vi "Factory.vi"(4 "Use LCD?":bool, 5 "Recycle?":bool, 6 "Reader":T2, 7 "Scan Setup Mode":T1, 8 "error in":errorcluster, 9 "Scanner":T3, 10 "Path":path, 11 "Recycle old Scan Driver in":refnum<class "Scan Driver.lvclass">) -> (0 "error out":errorcluster, 3 "Scan Driver out":refnum<class "Scan Driver.lvclass">)   [LabVIEW 2009, in "Scan Driver.lvclass"]
doc: "Construct a new Scan Driver instance using the given parameters, load one from a file, or recycle an old one."
uses:
  Scan Driver.lvclass
  Scanner List.ctl
  Reader List.ctl
  Scan Setup Mode.ctl
  Scan Driver.lvclass/Scan Driver.ctl
  Scanners/Scanner/Scanner.lvclass
  Instruments/Spectrometer/Spectrometer Triax 550.lvclass
  Instruments/Magnet/Power Supply/Power Supply.lvclass
  Instruments/Pulse Gen/Pulse Generator.lvclass
  Instruments/Function Generator/Function Generator.lvclass
  Instruments/Microwave/Microwave.lvclass
  Instruments/Translation Stages/Translation Stages.lvclass
  Instruments/Spectrometer Digikröm/Spectrometer Digikröm.lvclass
  Instruments/Spectrometer iHR320/Spectrometer iHR320.lvclass
  Instruments/Varian Magnet/Varian Magnet.lvclass
  Instruments/Analog Output/Analog Output.lvclass
  Instruments/Photon Counter/Photon Counter SR400.lvclass
  Instruments/Lockin/Lockin SR830.lvclass
  Instruments/Utility Classes/Dummy/Dummy.lvclass
  Instruments/DAQ/DAQmx Analog.lvclass
  Readers/Reader/Reader.lvclass
  Readers/PC Reader/PC Reader.lvclass
  File IO/File IO.lvclass
  Instruments/LCD/LCD Retarder.lvclass
  Readers/LCD Reader/LCD Reader.lvclass
  Scanners/Dummy Scan/Dummy Scan.lvclass
  Instruments/Magnet/Temperature Controller/Temperature Controller.lvclass
  Instruments/Fluke Multimeter/Fluke Multimeter.lvclass
  Instruments/Power Meter/Power Meter.lvclass
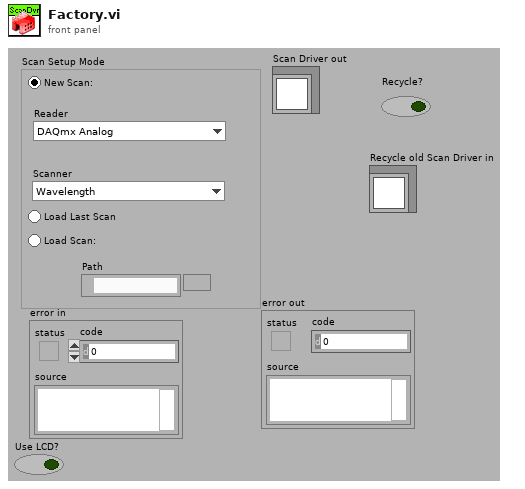
[diagram p1: front panel]
types:
  T1 = typedef "Scan Driver.lvclass/Scan Setup Mode.ctl" = enum32{"New Scan", "Load Last Scan", "Load Scan:"}
  T2 = typedef "Scan Driver.lvclass/Reader List.ctl" = enum16{"DAQmx Analog", "Dummy", "Lockin SR830", "Photon Counter", "Multimeter", "Power Meter", "Temperature Control"}
  T3 = typedef "Scan Driver.lvclass/Scanner List.ctl" = enum16{"Wavelength", "Wavelength Digikröm", "Wavelength iHR320", "Magnetic Field", "Continuous", "Pulse Gen Scan", "Pulse Gen Basic Scan", "Function Gen Scan", "Microwave Freq Scan", "Translation Stage Scan", "Dummy Scan", "Varian Magnet Scan", "Varian Continuous Scan", "Analog Output Scan"}
  T4 = typedef "Scanner.lvclass/Range.ctl" = cluster{"xi":dbl, "xf":dbl, "dx":dbl, "Return to...?":bool, "Return to":dbl}
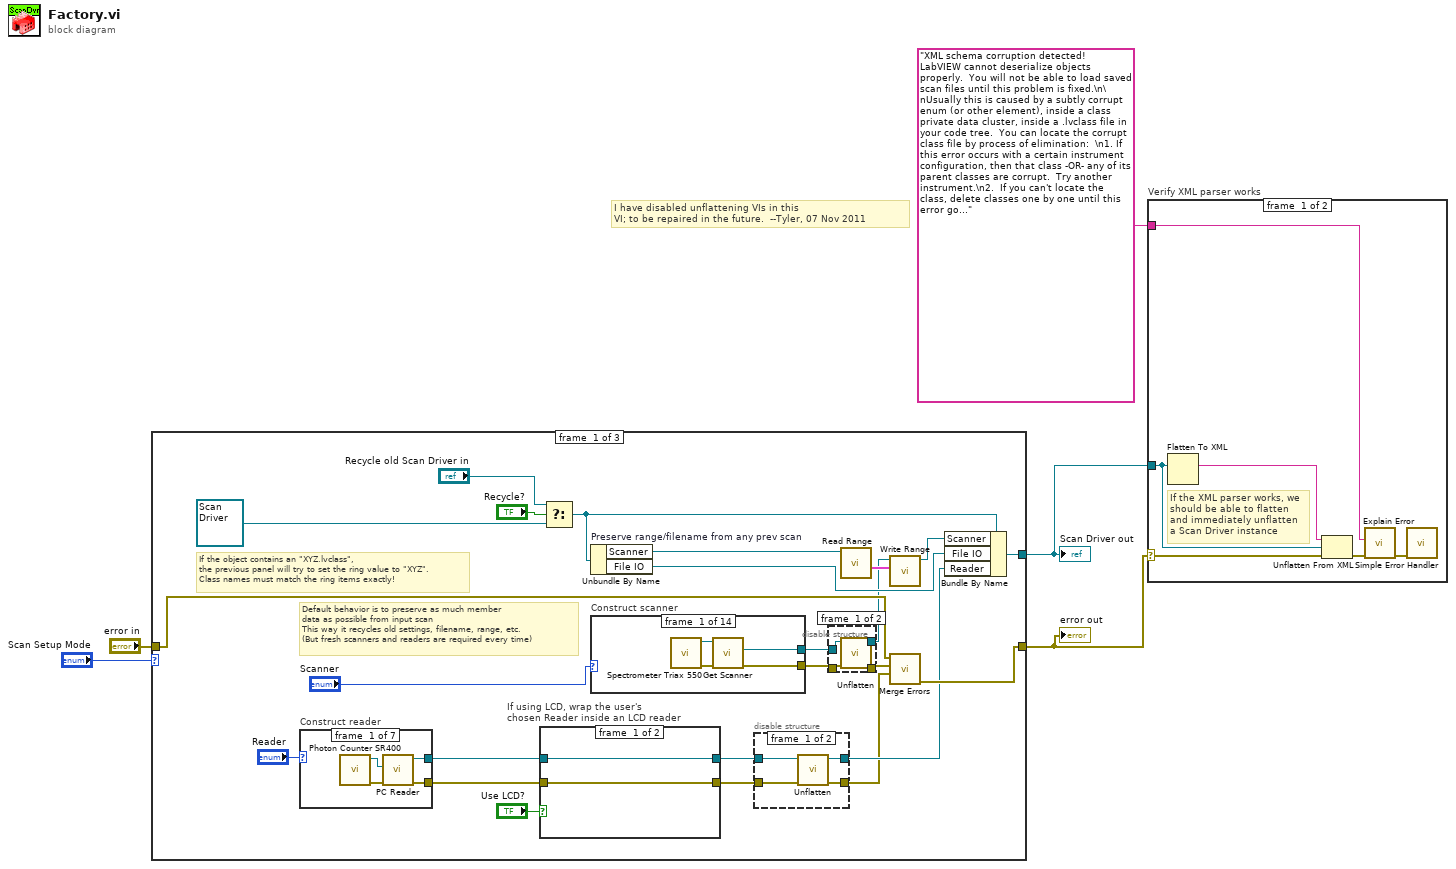
[diagram p0: block diagram]
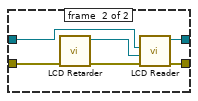
[diagram p5: hidden frame]
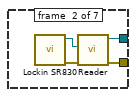
[diagram p6: hidden frame]
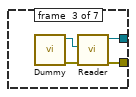
[diagram p7: hidden frame]
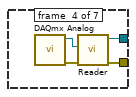
[diagram p8: hidden frame]
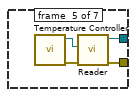
[diagram p9: hidden frame]
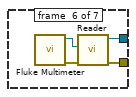
[diagram p10: hidden frame]
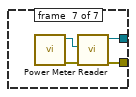
[diagram p11: hidden frame]
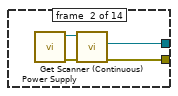
[diagram p12: hidden frame]
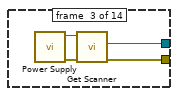
[diagram p13: hidden frame]
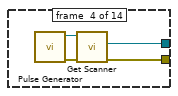
[diagram p14: hidden frame]
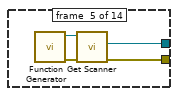
[diagram p15: hidden frame]
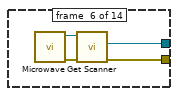
[diagram p16: hidden frame]
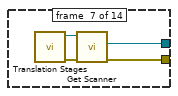
[diagram p17: hidden frame]
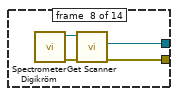
[diagram p18: hidden frame]
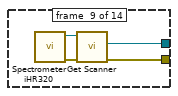
[diagram p19: hidden frame]
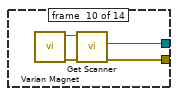
[diagram p20: hidden frame]
diagram:
  # "I have disabled unflattening VIs in this\nVI; to be repaired in the future.  --Tyler, 07 Nov 2011"
  n1 = case shown="\"New Scan\", Default" "Scan Setup Mode" {
    tunnel: [w29 w133 w138] -> w3
    tunnel: [w16 w134 w137] -> w1
    tunnel: "error in" -> [w17 w135 w136]
    frame #0 {
      # "Default behavior is to preserve as much member\ndata as possible from input scan\nThis way it recycles old settings, filename, range, etc.\n(But fresh scanners and readers are required every time)"
      # "If the object contains an \"XYZ.lvclass\",\nthe previous panel will try to set the ring value to \"XYZ\".\nClass names must match the ring items exactly!"
      n2 = case "Construct reader" shown="\"Lockin SR830\"" "Reader" {
        tunnel: [w52 w56 w60 w64 w69 w71 w75] -> w15
        tunnel: [w50 w54 w58 w62 w68 w70 w74] -> w13
        frame #0 {
          n3 = call "Photon Counter SR400.vi"() -> ("error out"=w51:errorcluster, "Photon Counter SR400 out"=w53:refnum<class "Photon Counter SR400.lvclass">)  [unwired: 10 out]
          n4 = call "PC Reader.vi"("error in (no error)"=w51, "Photon Counter SR400 in"=w53) -> ("error out"=w50:errorcluster, "PC Reader out"=w52:refnum<class "PC Reader.lvclass">)  [unwired: 8 out]
        }
        frame #1 {
          n5 = call "Lockin SR830.vi"() -> ("error out"=w55:errorcluster, "Lockin SR830 out"=w57:refnum<class "Lockin SR830.lvclass">)  [unwired: 1 in, 9 out]
          n6 = call "Reader.vi"("error in (no error)"=w55, "Readable"=w57) -> ("error out"=w54:errorcluster, "Reader out"=w56:refnum<class "Reader.lvclass">)  [unwired: 8 out]
        }
        frame #2 {
          n7 = call "Dummy.vi"() -> ("error out"=w59:errorcluster, "Dummy out"=w61:refnum<class "Dummy.lvclass">)  [unwired: 2 in, 8 out]
          n8 = call "Reader.vi"("error in (no error)"=w59, "Readable"=w61) -> ("error out"=w58:errorcluster, "Reader out"=w60:refnum<class "Reader.lvclass">)  [unwired: 8 out]
        }
        frame #3 {
          n9 = call "DAQmx Analog.vi"() -> ("error out"=w63:errorcluster, "DAQmx Analog out"=w65:refnum<class "DAQmx Analog.lvclass">)  [unwired: 1 in, 9 out]
          n10 = call "Reader.vi"("error in (no error)"=w63, "Readable"=w65) -> ("error out"=w62:errorcluster, "Reader out"=w64:refnum<class "Reader.lvclass">)  [unwired: 8 out]
        }
        frame #4 {
          n11 = call "Temperature Controller.vi"() -> ("error out"=w67:errorcluster, "Temperature Controller out"=w66:refnum<class "Temperature Controller.lvclass">)  [unwired: 10 in]
          n12 = call "Reader.vi"("error in (no error)"=w67, "Readable"=w66) -> ("error out"=w68:errorcluster, "Reader out"=w69:refnum<class "Reader.lvclass">)  [unwired: 8 out]
        }
        frame #5 {
          n13 = call "Fluke Multimeter.vi"() -> ("error out"=w73:errorcluster, "Fluke Multimeter out"=w72:refnum<class "Fluke Multimeter.lvclass">)  [unwired: 10 in]
          n14 = call "Reader.vi"("error in (no error)"=w73, "Readable"=w72) -> ("error out"=w70:errorcluster, "Reader out"=w71:refnum<class "Reader.lvclass">)  [unwired: 8 out]
        }
        frame #6 {
          n15 = call "Power Meter.vi"() -> ("error out"=w77:errorcluster, "Power Meter out"=w76:refnum<class "Power Meter.lvclass">)  [unwired: 10 in]
          n16 = call "Reader.vi"("error in (no error)"=w77, "Readable"=w76) -> ("error out"=w74:errorcluster, "Reader out"=w75:refnum<class "Reader.lvclass">)  [unwired: 8 out]
        }
      }
      n17 = case "If using LCD, wrap the user's \nchosen Reader inside an LCD reader" shown="True" "Use LCD?" {
        tunnel: w15 -> [w42 w46]
        tunnel: w13 -> [w43 w47]
        tunnel: [w43 w44] -> w7
        tunnel: [w42 w45] -> w14
        frame #0 {
        }
        frame #1 {
          n18 = call "LCD Retarder.vi"("error in"=w47) -> ("errorOUT"=w48:errorcluster, "LCD out"=w49:refnum<class "LCD Retarder.lvclass">)  [unwired: 9 out]
          n19 = call "LCD Reader.vi"("error in (no error)"=w48, "LCD Retarder in"=w49, "Reader.lvclass"=w46) -> ("error out"=w44:errorcluster, "LCD Reader out"=w45:refnum<class "LCD Reader.lvclass">)  [unwired: 2 in, 5 out]
        }
      }
      n20 = Select(t="Recycle old Scan Driver in", s="Recycle?", f=refnum<class "Scan Driver.lvclass"> refnum ("Recycle old Scan Driver in")) -> (s? t:f=w18:refnum<class "Scan Driver.lvclass">)
      n21 = Unbundle By Name "Preserve range/filename from any prev scan"(w18) -> ("Scanner"=w27:refnum<class "Scanner.lvclass">, "File IO"=w24:refnum<class "File IO.lvclass">)
      n22 = case "Construct scanner" shown="\"Microwave Freq Scan\"" "Scanner" {
        tunnel: [w80 w84 w88 w92 w96 w100 w104 w108 w110 w117 w118 w123 w127 w131] -> w28
        tunnel: [w79 w82 w86 w90 w94 w98 w102 w106 w111 w114 w119 w122 w126 w129] -> w9
        frame #0 {
          n23 = call "Spectrometer Triax 550.vi"() -> ("error out"=w78:errorcluster, "Spectrometer Triax 550 out"=w81:refnum<class "Spectrometer Triax 550.lvclass">)  [unwired: 2 in, 8 out]
          n24 = call-dynamic "Get Scanner.vi"("error in (no error)"=w78, "Spectrometer Triax 550 in"=w81) -> ("error out"=w79:errorcluster, "Default Scanner out"=w80:refnum<class "Scanner.lvclass">)  [unwired: 8 out]
        }
        frame #1 {
          n25 = call "Power Supply.vi"() -> ("error out"=w83:errorcluster, "Power Supply out"=w85:refnum<class "Power Supply.lvclass">)  [unwired: 10 in]
          n26 = call "Get Scanner (Continuous).vi"("error in (no error)"=w83, "Power Supply in"=w85) -> ("error out"=w82:errorcluster, "Continuous Scanner out"=w84:refnum<class "Continuous.lvclass">)  [unwired: 8 in]
        }
        frame #2 {
          n27 = call "Power Supply.vi"() -> ("error out"=w87:errorcluster, "Power Supply out"=w89:refnum<class "Power Supply.lvclass">)  [unwired: 10 in]
          n28 = call-dynamic "Get Scanner.vi"("error in (no error)"=w87, "Power Supply in"=w89) -> ("error out"=w86:errorcluster, "Default Scanner out"=w88:refnum<class "Scanner.lvclass">)  [unwired: 8 out]
        }
        frame #3 {
          n29 = call "Pulse Generator.vi"() -> ("error out"=w91:errorcluster, "Pulse Generator out"=w93:refnum<class "Pulse Generator.lvclass">)  [unwired: 1 in, 9 out]
          n30 = call-dynamic "Get Scanner.vi"("error in (no error)"=w91, "Pulse Generator in"=w93) -> ("error out"=w90:errorcluster, "Default Scanner out"=w92:refnum<class "Scanner.lvclass">)  [unwired: 8 out]
        }
        frame #4 {
          n31 = call "Function Generator.vi"() -> ("error out"=w95:errorcluster, "Function Generator out"=w97:refnum<class "Function Generator.lvclass">)  [unwired: 1 in, 9 out]
          n32 = call-dynamic "Get Scanner.vi"("error in (no error)"=w95, "Function Generator in"=w97) -> ("error out"=w94:errorcluster, "Default Scanner out"=w96:refnum<class "Scanner.lvclass">)  [unwired: 8 out]
        }
        frame #5 {
          n33 = call "Microwave.vi"() -> ("error out"=w99:errorcluster, "Microwave out"=w101:refnum<class "Microwave.lvclass">)  [unwired: 1 in, 9 out]
          n34 = call-dynamic "Get Scanner.vi"("error in (no error)"=w99, "Microwave in"=w101) -> ("error out"=w98:errorcluster, "Default Scanner out"=w100:refnum<class "Scanner.lvclass">)  [unwired: 8 out]
        }
        frame #6 {
          n35 = call "Translation Stages.vi"() -> ("error out"=w103:errorcluster, "Translation Stages out"=w105:refnum<class "Translation Stages.lvclass">)  [unwired: 1 in, 9 out]
          n36 = call-dynamic "Get Scanner.vi"("error in (no error)"=w103, "Translation Stages in"=w105) -> ("error out"=w102:errorcluster, "Default Scanner out"=w104:refnum<class "Scanner.lvclass">)  [unwired: 8 out]
        }
        frame #7 {
          n37 = call "Spectrometer Digikröm.vi"() -> ("error out"=w107:errorcluster, "Spectrometer Digikröm out"=w109:refnum<class "Spectrometer Digikröm.lvclass">)  [unwired: 1 in, 9 out]
          n38 = call-dynamic "Get Scanner.vi"("error in (no error)"=w107, "Spectrometer Digikröm in"=w109) -> ("error out"=w106:errorcluster, "Default Scanner out"=w108:refnum<class "Scanner.lvclass">)  [unwired: 8 out]
        }
        frame #8 {
          n39 = call "Spectrometer iHR320.vi"() -> ("error out"=w112:errorcluster, "Spectr. iHR320 Out"=w113:refnum<class "Spectrometer iHR320.lvclass">)  [unwired: 10 in]
          n40 = call-dynamic "Get Scanner.vi"("error in (no error)"=w112, "Spectrometer iHR320 in"=w113) -> ("error out"=w111:errorcluster, "Default Scanner out"=w110:refnum<class "Scanner.lvclass">)  [unwired: 8 in]
        }
        frame #9 {
          n41 = call "Varian Magnet.vi"() -> ("error out"=w115:errorcluster, "Varian Magnet out"=w116:refnum<class "Varian Magnet.lvclass">)  [unwired: 1 in, 9 out]
          n42 = call-dynamic "Get Scanner.vi"("error in (no error)"=w115, "Varian Magnet in"=w116) -> ("error out"=w114:errorcluster, "Default Scanner out"=w117:refnum<class "Scanner.lvclass">)  [unwired: 8 out]
        }
        frame #10 {
          n43 = call "Analog Output.vi"() -> ("error out"=w120:errorcluster, "Analog Output out"=w121:refnum<class "Analog Output.lvclass">)  [unwired: 10 in]
          n44 = call-dynamic "Get Scanner.vi"("error in (no error)"=w120, "Analog Output in"=w121) -> ("error out"=w119:errorcluster, "Default Scanner out"=w118:refnum<class "Scanner.lvclass">)  [unwired: 8 in]
        }
        frame #11 {
          n45 = call "Pulse Generator.vi"() -> ("error out"=w124:errorcluster, "Pulse Generator out"=w125:refnum<class "Pulse Generator.lvclass">)  [unwired: 1 in, 9 out]
          n46 = call-dynamic "Get Scanner (basic).vi"("error in (no error)"=w124, "Pulse Generator in"=w125) -> ("error out"=w122:errorcluster, "Pulse Gen Basic Scanner out"=w123:refnum<class "Scanner.lvclass">)  [unwired: 8 in]
        }
        frame #12 {
          n47 = call "Dummy Scan.vi"() -> ("error out"=w126:errorcluster, "Dummy Scan out"=w127:refnum<class "Dummy Scan.lvclass">)  [unwired: 10 in]
        }
        frame #13 {
          n48 = call "Varian Magnet.vi"() -> ("error out"=w130:errorcluster, "Varian Magnet out"=w128:refnum<class "Varian Magnet.lvclass">)  [unwired: 1 in, 9 out]
          n49 = call "Get Scanner (continuous).vi"("error in (no error)"=w130, "Varian Magnet.lvclass"=w128) -> ("error out"=w129:errorcluster, "Default Scanner out"=w131:refnum<class "Scanner.lvclass">)  [unwired: 8 in]
        }
      }
      n50 = disable-structure shown="Enabled" {
        disable-tunnel: w14 -> [w39 w40]
        disable-tunnel: [w38 w40] -> w8
        disable-tunnel: w7 -> [w37 w41]
        disable-tunnel: [w36 w41] -> w6
        frame #0 {
          n51 = call-dynamic "Unflatten.vi"("error in (no error)"=w37, "Reader in"=w39) -> ("error out"=w36:errorcluster, "Reader out"=w38:refnum<class "Reader.lvclass">)  [unwired: 8 in]
        }
        frame #1 {
        }
      }
      n52 = disable-structure shown="Enabled" {
        disable-tunnel: w28 -> [w33 w35]
        disable-tunnel: [w32 w35] -> w11
        disable-tunnel: [w31 w34] -> w10
        disable-tunnel: w9 -> [w30 w34]
        frame #0 {
          n53 = call-dynamic "Unflatten.vi"("error in (no error)"=w30, "Scanner in"=w33) -> ("error out"=w31:errorcluster, "Scanner out"=w32:refnum<class "Scanner.lvclass">)  [unwired: 8 in]
        }
        frame #1 {
        }
      }
      n54 = call-dynamic "Read Range.vi"("Scanner.lvclass in"=w27) -> ("Range"=w25:T4)  [unwired: 1 in, 9 out]
      n55 = call-dynamic "Write Range.vi"("Range"=w25, "Scanner in"=w11) -> ("Scanner out"=w26:refnum<class "Scanner.lvclass">)  [unwired: 1 in, 8 out]
      n56 = call <vilib>:"Merge Errors.vi"("error in 3 (no error)"=w6, "error in 2 (no error)"=w10, "error in 1 (no error)"=w17) -> ("error out"=w16:errorcluster)  [unwired: 1 in, 3 out]
      n57 = Bundle By Name(cluster=w18, "Scanner"=w26, "File IO"=w24, "Reader"=w8) -> (w29:refnum<class "Scan Driver.lvclass">)
    }
    frame #1 {
      n58 = call "Load Scan.vi"("error in (no error)"=w135, "XML File Path"="Path") -> ("error out"=w134:errorcluster, "Scan Driver out"=w133:refnum<class "Scan Driver.lvclass">)  [unwired: 8 out]
    }
    frame #2 {
      n59 = call "Load Last Scan.vi"("error in"=w136) -> ("error out"=w137:errorcluster, "Last Run Scan"=w138:refnum<class "Scan Driver.lvclass">)  [unwired: 9 out]
    }
  }
  "error out" <- w1
  "Scan Driver out" <- w3
  n60 = case "Verify XML parser works" shown="No Error" w1 {
    selector: w1 -> [w143 _]
    tunnel: w3 -> [w139 _]
    tunnel: "XML schema corruption detected!  LabVIEW cannot deserialize objects properly.  You will not be able to load saved scan files until this problem is fixed.\n\nUsually this is caused by a subtly corrupt enum (or other element), inside a class private data cluster, inside a .lvclass file in your code tree.  You can locate the corrupt class file by process of elimination:  \n1. If this error occurs with a certain instrument configuration, then that class -OR- any of its parent classes are corrupt.  Try another instrument.\n2.  If you can't locate the class, delete classes one by one until this error goes away.\nOnce you find the offending class:\n3. Replace all enums in the class data cluster with rings.\n4. Try to roll back the class file with Subversion.\n5. If all else fails, delete all elements of its private data cluster one by one until the problem goes away.  Then recreate each element by hand (not by copy-pasting.)" -> [w141 _]
    frame #0 {
      # "If the XML parser works, we \nshould be able to flatten\nand immediately unflatten\na Scan Driver instance"
      n61 = Flatten To XML(anything=w139) -> (xml string=w144:string)
      n62 = Unflatten From XML(xml string=w144, type=w139, error in (no error)=w143) -> (error out=w142:errorcluster)  [unwired: 1 out]
      n63 = call "Explain Error.vi"("error in"=w142, "Explanation"=w141) -> ("error out"=w140:errorcluster)  [unwired: 9 out]
      n64 = call <vilib>:"Simple Error Handler.vi"("error in (no error)"=w140) -> ()  [unwired: 1 in, 8 out]
    }
    frame #1 {
    }
  }
